vi "CalculateTau.vi"(1 "g2 data":sgl[](array[numeric]), 2 "delaytime":sgl[](array[numeric]), 3 "array size":i32) -> (0 "Tau":sgl)   [LabVIEW 2011]
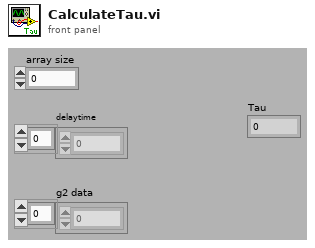
[diagram p1: front panel]
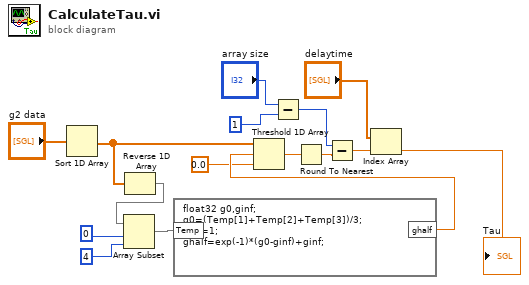
[diagram p0: block diagram]
diagram:
  n1 = Sort 1D Array(array="g2 data") -> (sorted array=w7:sgl[])
  n2 = Reverse 1D Array(array=w7) -> (reversed array=w6:sgl[])
  n3 = Array Subset(array=w6, index=0, length=4) -> (w14:sgl[])
  n4 = formula code="float32 g0,ginf;\ng0=(Temp[1]+Temp[2]+Temp[3])/3;\nginf=1;\nghalf=exp(-1)*(g0-ginf)+ginf;"("Temp"=w14) -> ("ghalf"=w11:dbl)
  n5 = Threshold 1D Array(1:sgl 0.0, 2:w11, 3:w7) -> (0:w5:sgl)
  n6 = Subtract(x="array size", y=1) -> (x-y=w12:i32)
  n7 = Round To Nearest(number=w5) -> (nearest integer value=w4:sgl)
  n8 = Subtract(x=w12, y=w4) -> (x-y=w1:sgl)
  n9 = Index Array(array="delaytime", index=w1) -> (element=→"Tau":sgl)
